vi "Adjust Target Focus.vi"(0 "Target":T3, 1 "System of Reference Interface":T5, 2 "Focus and Tracking":T4, 3 "Calibration":T1, 5 "error in (no error)":errorcluster, 6 "Distance [um]":dbl=100.0, 7 "Frames per plane [unused]":i32=3, 8 "Refocus Step [um]":dbl=1.0, 10 "Z direction":i8(ring)=-1 items=["Positive"=1, "Negative"=-1], 13 "Active":refnum<vi>) -> (12 "CFS":dbl, 14 "Focus Failed":bool, 15 "Estimated Coordinates [um]":T2, 16 "Actual Coordinates [um]":T2, 17 "Aborted":bool, 18 "Scope Error":bool, 19 "error out":errorcluster)   [LabVIEW 2012, in "Targeting Unit.lvlib"]
uses:
  Targeting Unit.lvlib
  <vilib>/Analysis/Matrix/Datatypes/RealMatrix.ctl
  <vilib>/Analysis/NI_AALPro.lvlib
  <vilib>/Analysis/Matrix/NI_Matrix.lvlib
panel:
  out "Depth[um]":dbl
  out "standard deviation":dbl
  out "center":dbl
  out "Observed Data and Fitted Curve":cluster{cluster{dbl, "Numeric":dbl}[]}[](graph)
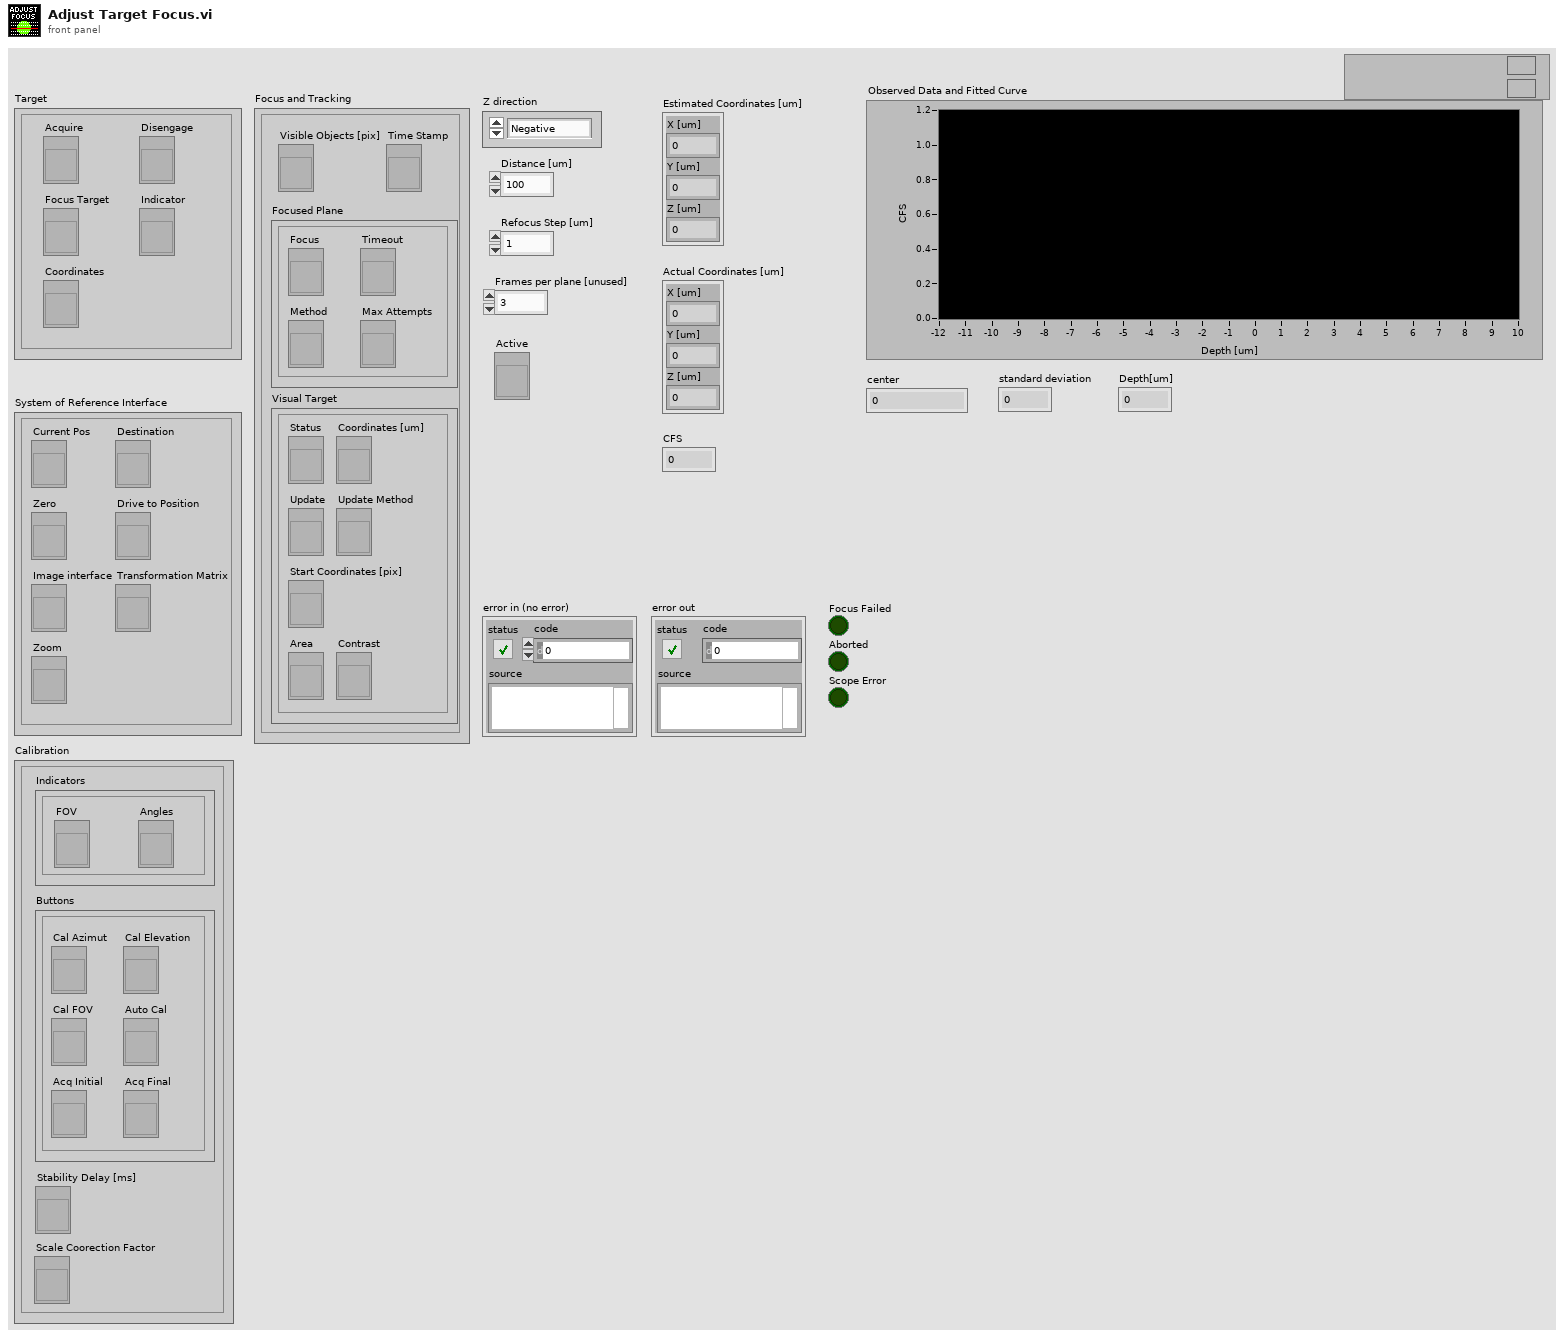
[diagram p1: front panel]
types:
  T1 = cluster{"Indicators":cluster{"FOV":refnum<vi>, "Angles":refnum<vi>}, "Buttons":cluster{"Cal FOV":refnum<vi>, "Cal Azimut":refnum<vi>, "Cal Elevation":refnum<vi>, "Auto Cal":refnum<vi>, "Acq Initial":refnum<vi>, "Acq Final":refnum<vi>}, "Stability Delay [ms]":refnum<vi>, "Scale Coorection Factor":refnum<vi>}
  T2 = cluster{"X [um]":dbl, "Y [um]":dbl, "Z [um]":dbl}
  T3 = cluster{"Coordinates":refnum<vi>, "Acquire":refnum<vi>, "Disengage":refnum<vi>, "Indicator":refnum<vi>, "Focus Target":refnum<vi>}
  T4 = cluster{"Focused Plane":cluster{"Focus":refnum<vi>, "Timeout":refnum<vi>, "Max Attempts":refnum<vi>, "Method":refnum<vi>}, "Time Stamp":refnum<vi>, "Visual Target":cluster{"Coordinates [um]":refnum<vi>, "Status":refnum<vi>, "Update":refnum<vi>, "Update Method":refnum<vi>, "Start Coordinates [pix]":refnum<vi>, "Area":refnum<vi>, "Contrast":refnum<vi>}, "Visible Objects [pix]":refnum<vi>}
  T5 = cluster{"Current Pos":refnum<vi>, "Image interface":refnum<vi>, "Transformation Matrix":refnum<vi>, "Zero":refnum<vi>, "Destination":refnum<vi>, "Drive to Position":refnum<vi>, "Zoom":refnum<vi>}
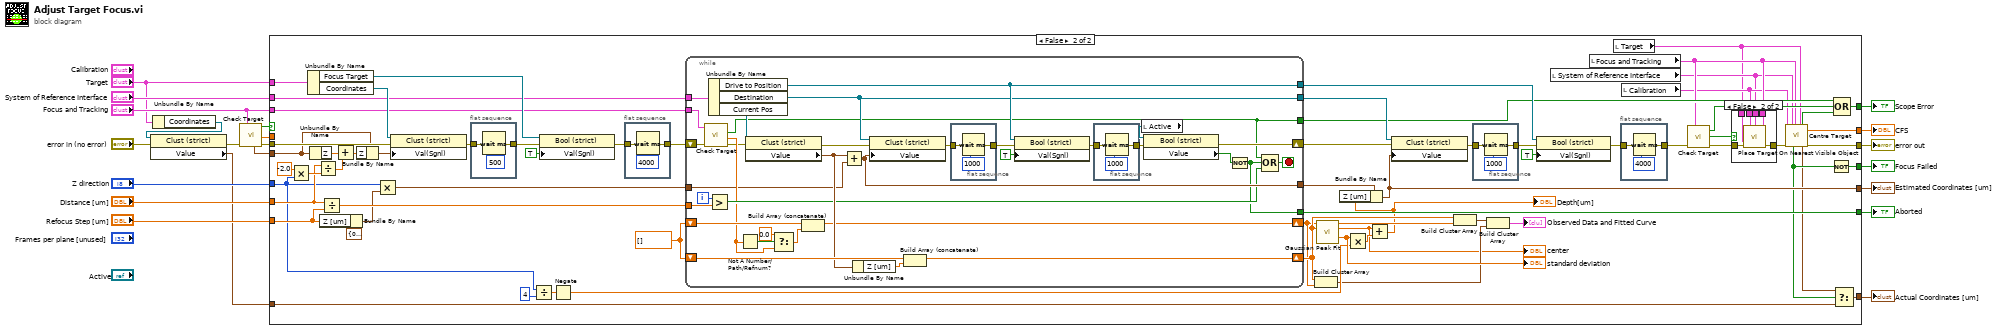
[diagram p0: block diagram]
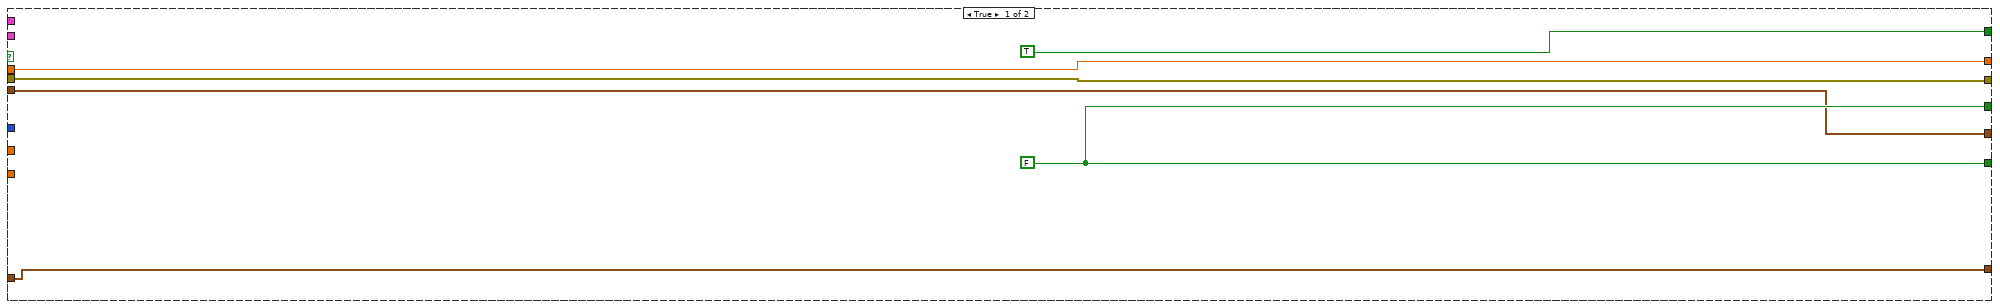
[diagram p2: hidden frame]
diagram:
  n1 = Unbundle By Name("Target") -> ("Coordinates"=w6:refnum<vi>)
  n2 = property class="Clust (strict)"(reference=w6, error in="error in (no error)") -> (error out=w7:errorcluster, "Value"=w4:T2)  [unwired: 1 out]
  n3 = call "Check Target.vi"("Error In"=w7, "Focus and Tracking"="Focus and Tracking") -> ("Error out"=w16:errorcluster, "CFS"=w1:dbl, "Scope Error"=w12:bool, "Optical Coordinates [um]"=w14:cluster{"X":dbl, "Y":dbl, "Z":dbl})  [unwired: 3 in, 3 out]
  n4 = case shown="False" w12 {
    tunnel: "Distance [um]" -> [_ w65]
    tunnel: [w24 w54] -> w20
    tunnel: [w26 w80] -> w19
    tunnel: "System of Reference Interface" -> [_ w79]
    tunnel: "Target" -> [_ w78]
    tunnel: [w25 w36] -> w17
    tunnel: [TRUE w38] -> w10
    tunnel: w16 -> [w25 w76]
    tunnel: "Focus and Tracking" -> [_ w75]
    tunnel: w14 -> [w24 w74]
    tunnel: "Refocus Step [um]" -> [_ w73]
    tunnel: "Z direction" -> [_ w47]
    tunnel: [w26 w69] -> w9
    tunnel: w4 -> [w23 w64]
    tunnel: [w23 w63] -> w3
    tunnel: [w22 w35] -> w2
    tunnel: w1 -> [w22 _]
    frame True {
      w26 = FALSE ("Value")
    }
    frame False {
      w81 = dbl[] []
      n5 = Multiply(x=-2.0 ("y"), y=w47) -> (x*y=w67:dbl)
      n6 = Unbundle By Name(w78) -> ("Focus Target"=w91:refnum<vi>, "Coordinates"=w92:refnum<vi>)
      n7 = Unbundle By Name(w74) -> ("Z"=w89:dbl)
      n8 = Divide(x=w65, y=w67) -> (x/y=w87:dbl)
      n9 = Bundle By Name(cluster=T2 {"X [um]"=0.0, "Y [um]"=0.0, "Z [um]"=0.0} ("y"), "Z [um]"=w73) -> (w70:T2)
      n10 = Divide(x=w65, y=w73) -> (x/y=w95:dbl)
      n11 = Add(x=w89, y=w87) -> (x+y=w88:dbl)
      n12 = Bundle By Name(cluster=w74, "Z"=w88) -> (w90:cluster{"X":dbl, "Y":dbl, "Z":dbl})
      n13 = Multiply(x=w47, y=w70) -> (x*y=w71:T2)
      n14 = property class="Clust (strict)"(reference=w92, error in=w76, "Val(Sgnl)"=w90) -> (error out=w94:errorcluster)  [unwired: 1 out]
      n15 = flat-sequence {
        tunnel: [w110] -> w93
        tunnel: w94 -> [w110]
        frame #0 {
          n16 = Wait (ms)(milliseconds to wait=u32 500) -> ()  [unwired: 1 out]
        }
      }
      n17 = Divide(x=w47, y=i8 4) -> (x/y=w46:dbl)
      n18 = property class="Bool (strict)"(reference=w91, error in=w93, "Val(Sgnl)"=TRUE ("Value (Signaling)")) -> (error out=w59:errorcluster)  [unwired: 1 out]
      n19 = Negate(x=w46) -> (-x=w50:dbl)
      n20 = flat-sequence {
        tunnel: [w104] -> w58
        tunnel: w59 -> [w104]
        frame #0 {
          n21 = Wait (ms)(milliseconds to wait=u32 4000) -> ()  [unwired: 1 out]
        }
      }
      n22 = while {
        shift-right: [w142] -> w84
        shift-left: w58 -> [w119]
        shift-right: [w113] -> w55
        shift-left: w81 -> [w144]
        tunnel: w75 -> [w120]
        tunnel: w95 -> [w141]
        tunnel: [w116] -> w40
        shift-right: [w114] -> w57
        shift-left: w81 -> [w130]
        tunnel: [w127] -> w83
        tunnel: [w126] -> w82
        tunnel: [w125] -> w68
        tunnel: w79 -> [w124]
        tunnel: [w111] -> w80
        tunnel: w71 -> [w117]
        i -> [w140]
        stop <- w143 stop-if-true
        n23 = call "Check Target.vi"("Error In"=w119, "Focus and Tracking"=w120) -> ("Error out"=w118:errorcluster, "CFS"=w121:dbl, "Scope Error"=w116:bool)  [unwired: 3 in, 4 out]
        n24 = Unbundle By Name(w124) -> ("Drive to Position"=w127:refnum<vi>, "Destination"=w126:refnum<vi>, "Current Pos"=w136:refnum<vi>)
        n25 = Greater?(x=w140, y=w141) -> (0:w122:bool)
        n26 = Not A Number/Path/Refnum?(number/path/refnum=w121) -> (NaN/Path/Refnum?=w133:bool)
        n27 = property class="Clust (strict)"(reference=w136, error in=w118) -> (error out=w135:errorcluster, "Value"=w129:T2)  [unwired: 1 out]
        n28 = Select(t=0.0, s=w133, f=w121) -> (s? t:f=w131:dbl)
        n29 = Build Array (concatenate)(w144, w131) -> (w113:dbl[])
        n30 = Add(x=w129, y=w117) -> (x+y=w125:T2)
        n31 = Unbundle By Name(w129) -> ("Z [um]"=w128:dbl)
        n32 = property class="Clust (strict)"(reference=w126, error in=w135, "Value"=w125) -> (error out=w137:errorcluster)  [unwired: 1 out]
        n33 = Build Array (concatenate)(w130, w128) -> (w114:dbl[])
        n34 = flat-sequence {
          tunnel: [w148] -> w138
          tunnel: w137 -> [w148]
          frame #0 {
            n35 = Wait (ms)(milliseconds to wait=u32 1000) -> ()  [unwired: 1 out]
          }
        }
        n36 = property class="Bool (strict)"(reference=w127, error in=w138, "Val(Sgnl)"=TRUE ("Value")) -> (error out=w139:errorcluster)  [unwired: 1 out]
        n37 = flat-sequence {
          tunnel: [w146] -> w134
          tunnel: w139 -> [w146]
          frame #0 {
            n38 = Wait (ms)(milliseconds to wait=u32 1000) -> ()  [unwired: 1 out]
          }
        }
        n39 = local read "Active"() -> (w112:refnum<vi>)
        n40 = property class="Bool (strict)"(reference=w112, error in=w134) -> (error out=w142:errorcluster, "Value"=w123:bool)  [unwired: 1 out]
        n41 = Not(x=w123) -> (.not. x?=w111:bool)
        n42 = Compound Arithmetic op=OR(w116, w111, w122) -> (w143:bool)
      }
      n43 = Build Cluster Array(w57, w55) -> (w45:cluster{"Value":dbl, "Value":dbl}[])
      n44 = call <vilib>:"Gaussian Peak Fit.vi"("Y"=w55, "X"=w57) -> ("Best Gaussian Fit"=w56:dbl[], "center"=w44:dbl, "standard deviation"=w52:dbl)  [unwired: 7 in, 4 out]
      "center" <- w44
      "standard deviation" <- w52
      n45 = Multiply(x=w52, y=w50) -> (x*y=w51:dbl)
      n46 = Add(x=w44, y=w51) -> (x+y=w49:dbl)
      "Depth[um]" <- w49
      n47 = Bundle By Name(cluster=w68, "Z [um]"=w49) -> (w54:T2)
      n48 = property class="Clust (strict)"(reference=w82, error in=w84, "Value"=w54) -> (error out=w86:errorcluster)  [unwired: 1 out]
      n49 = Build Cluster Array(w57, w56) -> (w62:cluster{"Value":dbl, "Numeric":dbl}[])
      n50 = flat-sequence {
        tunnel: [w108] -> w85
        tunnel: w86 -> [w108]
        frame #0 {
          n51 = Wait (ms)(milliseconds to wait=u32 1000) -> ()  [unwired: 1 out]
        }
      }
      n52 = Build Cluster Array(w62, w45) -> (→"Observed Data and Fitted Curve":cluster{cluster{"Value":dbl, "Value":dbl}[]}[])
      n53 = property class="Bool (strict)"(reference=w83, error in=w85, "Val(Sgnl)"=TRUE ("Value")) -> (error out=w77:errorcluster)  [unwired: 1 out]
      n54 = local read "System of Reference Interface"() -> (w29:T5)
      n55 = local read "Focus and Tracking"() -> (w31:T4)
      n56 = local read "Target"() -> (w28:T3)
      n57 = flat-sequence {
        tunnel: [w106] -> w43
        tunnel: w77 -> [w106]
        frame #0 {
          n58 = Wait (ms)(milliseconds to wait=u32 4000) -> ()  [unwired: 1 out]
        }
      }
      n59 = local read "Calibration"() -> (w30:T1)
      n60 = call "Check Target.vi"("Error In"=w43, "Focus and Tracking"=w31) -> ("Error out"=w42:errorcluster, "Scope Error"=w39:bool, "Target OK"=w41:bool)  [unwired: 3 in, 4 out]
      n61 = case shown="False" w41 {
        tunnel: [w96 w102] -> w37
        tunnel: w31 -> [_ w101]
        tunnel: w29 -> [_ w100]
        tunnel: w30 -> [_ w99]
        tunnel: w42 -> [w96 w98]
        tunnel: w28 -> [_ w97]
        frame True {
        }
        frame False {
          n62 = call "Place Target On Nearest Visible Object.vi"("Focus and Tracking"=w101, "System of Reference Interface"=w100, "Calibration"=w99, "Target"=w97, "error in (no error)"=w98) -> ("error out"=w102:errorcluster)  [unwired: 9 in, 1 out]
        }
      }
      n63 = call "Centre Target.vi"("Focus and Tracking"=w31, "Calibration"=w30, "System of Reference Interface"=w29, "Target"=w28, "error in (no error)"=w37) -> ("CFS"=w35:dbl, "Optical Coordinates [um]"=w32:cluster{"X":dbl, "Y":dbl, "Z":dbl}, "Scope Error"=w34:bool, "Target OK"=w33:bool, "error out"=w36:errorcluster)  [unwired: 8 in, 2 out]
      n64 = Not(x=w33) -> (.not. x?=w69:bool)
      n65 = Select(t=w32, s=w33, f=w64) -> (s? t:f=w63:T2)
      n66 = Compound Arithmetic op=OR(w40, w39, w34) -> (w38:bool)
    }
  }
  "Focus Failed" <- w9
  "Aborted" <- w19
  "Scope Error" <- w10
  "error out" <- w17
  "Estimated Coordinates [um]" <- w20
  "Actual Coordinates [um]" <- w3
  "CFS" <- w2
